vi "NI VeriStand - Get Multiple Dependent Node Refs.vi"(8 "error in (no error)":errorcluster, 10 "Base Property Name":string, 11 "Item Ref in":T1 format="%.0x") -> (0 "error out":errorcluster, 1 "Dependent Node Refs":T1[](array[typedef]) format="%.0x", 3 "Item Ref out":T1=18446744073709551615 format="%.0x")   [LabVIEW 2020, in "Custom Device Utility Library.lvlib"]
doc: "Gets the dependent node references that are set as values for properties of an item you specify. Dependent node references map to other nodes in the custom device, such as channels from which properties get their values. \n\nAll the properties must share the same base name. This VI increments a decimal appended to the <B>Base Property Name</B> until it cannot find any more properties."
uses:
  <vilib>/NI VeriStand/Custom Device Tools/Custom Device Utility Library/Custom Device Utility Library.lvlib
  <vilib>/NI VeriStand/Custom Device API/Custom Device Item Ref.ctl
  <vilib>/NI VeriStand/Custom Device API/Get Item Property (Dependent Node Pointer).vi
  <vilib>/NI VeriStand/Custom Device API/Custom Device API.lvlib
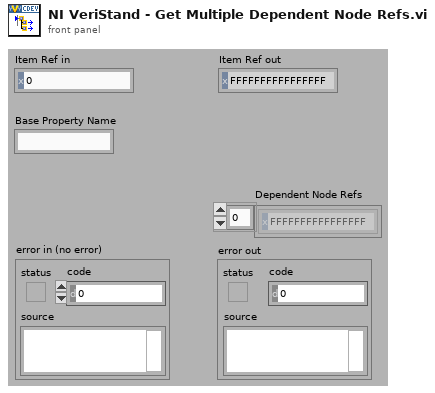
[diagram p1: front panel]
types:
  T1 = typedef "Custom Device API.lvlib/Custom Device Item Ref.ctl" = u64
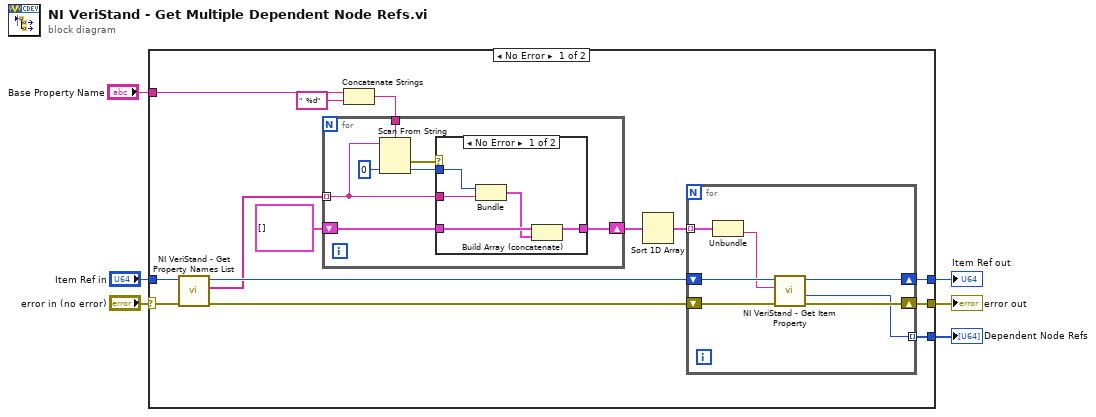
[diagram p0: block diagram]
diagram:
  n1 = case shown="No Error" "error in (no error)" {
    selector: "error in (no error)" -> [w16 w41]
    tunnel: "Item Ref in" -> [w20 w42]
    tunnel: [w11 w42] -> w5
    tunnel: [w10 w41] -> w4
    tunnel: "Base Property Name" -> [w19 _]
    tunnel: [w8 _] -> w1
    frame No Error {
      n2 = call <vilib>:"NI VeriStand - Get Property Names List.vi"("error in (no error)"=w16, "Item Ref in"=w20) -> ("error out"=w12:errorcluster, "Property Names"=w7:string[], "Item Ref out"=w13:T1)  [unwired: 7 in]
      n3 = Concatenate Strings(w19, "  %d" ("string")) -> (w17:string)
      n4 = for {
        tunnel: w7 -> [w33] mode=indexing
        tunnel: w17 -> [w32]
        shift-right: [w29] -> w14
        shift-left: cluster{"default value 1":i32, string}[] [] -> [w28]
        n5 = Scan From String(format string=w32, input string=w33, default 1=0 ("default value 1")) -> (error out=w34:errorcluster, output 1=w30:i32)  [unwired: 2 in, 2 out]
        n6 = case shown="No Error" w34 {
          tunnel: w33 -> [w38 _]
          tunnel: w30 -> [w39 _]
          tunnel: [w37 w40] -> w29
          tunnel: w28 -> [w36 w40]
          frame No Error {
            n7 = Bundle("default value 1"=w39, w38) -> (w35:cluster{"default value 1":i32, string})  [unwired: 1 in]
            n8 = Build Array (concatenate)(w36, w35) -> (w37:cluster{"default value 1":i32, string}[])
          }
          frame Error {
          }
        }
      }
      n9 = Sort 1D Array(array=w14) -> (sorted array=w9:cluster{"default value 1":i32, string}[])
      n10 = for {
        shift-right: [w25] -> w11
        shift-left: w13 -> [w27]
        shift-right: [w24] -> w10
        shift-left: w12 -> [w26]
        tunnel: w9 -> [w23] mode=indexing
        tunnel: [w21] -> w8 mode=indexing
        n11 = Unbundle(w23) -> (w22:string)  [unwired: 1 out]
        n12 = call-poly <vilib>:"NI VeriStand - Get Item Property.vi"("error in (no error)"=w26, "Property Name"=w22, "Item Ref in"=w27) -> ("error out"=w24:errorcluster, "Dependent Node Ref"=w21:T1, "Item Ref out"=w25:T1)  [unwired: 5 in, 1 out]
      }
    }
    frame Error {
    }
  }
  "Dependent Node Refs" <- w1
  "Item Ref out" <- w5
  "error out" <- w4
